vi "Exercise_Caculator.vi"() -> ()   [LabVIEW 2017]
panel:
  in  "stop":bool
  in  "Operations":T1(ring)
  out "Answer":dbl
  in  "Input 2":dbl
  in  "Input 1":dbl
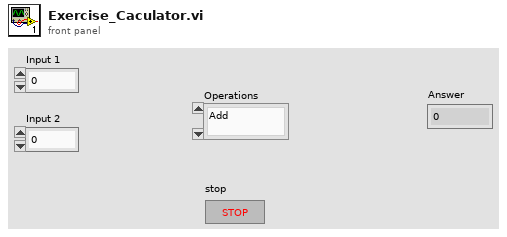
[diagram p1: front panel]
types:
  T1 = enum16{"Add", "Subtract", "Multiply", "Divide", "Square", "SquareRoot"}
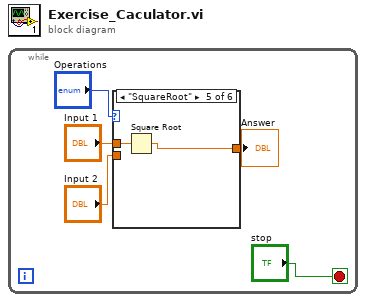
[diagram p0: block diagram]
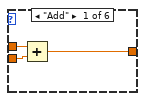
[diagram p2: hidden frame]
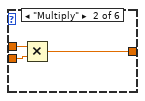
[diagram p3: hidden frame]
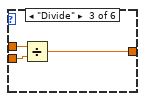
[diagram p4: hidden frame]
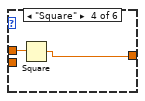
[diagram p5: hidden frame]
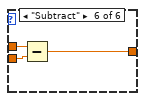
[diagram p6: hidden frame]
diagram:
  n1 = while {
    stop <- "stop" stop-if-true
    n2 = case shown="\"SquareRoot\"" "Operations" {
      tunnel: "Input 2" -> [w7 w10 w13 _ _ w20]
      tunnel: "Input 1" -> [w8 w11 w14 w15 w17 w21]
      tunnel: [w6 w9 w12 w16 w18 w19] -> w3
      frame "Add" {
        n3 = Add(x=w8, y=w7) -> (x+y=w6:dbl)
      }
      frame "Multiply" {
        n4 = Multiply(x=w11, y=w10) -> (x*y=w9:dbl)
      }
      frame "Divide" {
        n5 = Divide(x=w14, y=w13) -> (x/y=w12:dbl)
      }
      frame "Square" {
        n6 = Square(x=w15) -> (x^2=w16:dbl)
      }
      frame "SquareRoot" {
        n7 = Square Root(x=w17) -> (sqrt(x)=w18:dbl)
      }
      frame "Subtract" {
        n8 = Subtract(x=w21, y=w20) -> (x-y=w19:dbl)
      }
    }
    "Answer" <- w3
  }
